vi "Get IPs.vi"(11 "configuration file path":path=path "C:/UTP/config/Configuration.ini") -> (2 "Devices":string[](array[string]), 3 "IPs":string[](array[string]))   [LabVIEW 2025]
uses:
  <vilib>/Utility/config.llb/Read Key (String).vi
  <vilib>/Utility/config.llb/NI_LVConfig.lvlib
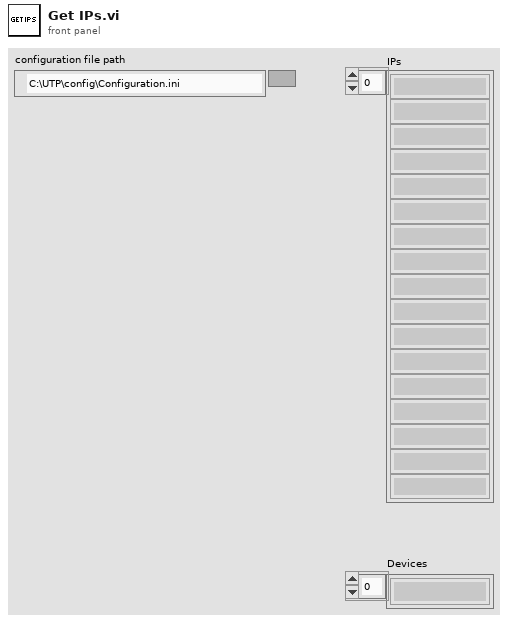
[diagram p1: front panel]
types:
  T1 = typedef "NI_LVConfig.lvlib/Config Data RefNum.ctl" = refnum<k1>
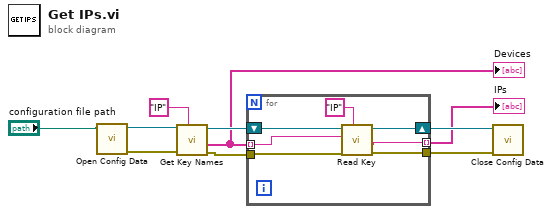
[diagram p0: block diagram]
diagram:
  n1 = call <vilib>:"Open Config Data.vi"("configuration file path"="configuration file path") -> ("error out"=w6:errorcluster, "refnum"=w9:T1)  [unwired: 8 in, 1 out]
  n2 = call <vilib>:"Get Key Names.vi"("section"="IP", "error in (no error)"=w6, "refnum"=w9) -> ("error out"=w5:errorcluster, "key names"=w1:string[], "refnum out"=w8:T1)  [unwired: 5 in, 1 out]
  "Devices" <- w1
  n3 = for {
    shift-right: [w16] -> w7
    shift-left: w8 -> [w17]
    tunnel: w1 -> [w15] mode=indexing
    tunnel: w5 -> [w14]
    tunnel: [w13] -> w4
    tunnel: [w12] -> w3 mode=indexing
    n4 = call-poly <vilib>:"Read Key.vi"("section"="IP", "error in (no error)"=w14, "key"=w15, "refnum"=w17) -> ("error out"=w13:errorcluster, "value"=w12:string, "refnum out"=w16:T1)  [unwired: 4 in, 1 out]
  }
  "IPs" <- w3
  n5 = call <vilib>:"Close Config Data.vi"("error in (no error)"=w4, "refnum"=w7) -> ()  [unwired: 8 in, 2 out]
